vi "Call DQMH Get Event Info VI QD.vi"(8 "error in (no error)":errorcluster, 11 "ProjectItem in":refnum<vi>) -> (0 "error out":errorcluster, 2 "Event Name":string, 4 "VI Ref":refnum<vi>)   [LabVIEW 2017]
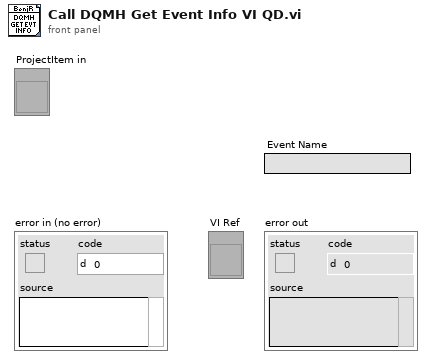
[diagram p1: front panel]
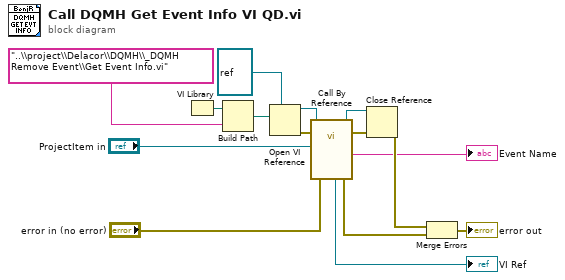
[diagram p0: block diagram]
diagram:
  n1 = VI Library() -> (path=w12:path)
  n2 = Build Path(base path=w12, name or relative path="..\\project\\Delacor\\DQMH\\_DQMH Remove Event\\Get Event Info.vi") -> (appended path=w11:path)
  n3 = Open VI Reference(type specifier VI Refnum (for type only)=refnum<vi> refnum, vi path=w11) -> (vi reference=w15:refnum<vi>, error out=w7:errorcluster)  [unwired: 4 in]
  n4 = call-by-ref "?"(reference=w15, error in=w7, 8:"error in (no error)"="error in (no error)", "ProjectItem in"="ProjectItem in") -> (reference out=w13:refnum<vi>, error out=w14:errorcluster, 0:"error out"=w10:errorcluster, "Event Name"=→"Event Name":string, "VI Ref"=→"VI Ref":refnum<vi>)  [unwired: 5 in, 2 out]
  n5 = Close Reference(reference=w13, error in (no error)=w14) -> (error out=w9:errorcluster)
  n6 = Merge Errors(w9, w10) -> (→"error out":errorcluster)
